vi "1D Explorer.vi"() -> ()   [LabVIEW 2023]
doc: "Demonstrates how to find the roots, maxima, and minima points for an equation entered on the front panel. This example also finds the integral and derivative for the equation."
uses:
  <vilib>/gmath/NI_Gmath.lvlib
panel:
  in  "Graph Options":i32[](listbox)
  out "Graph":cluster{dbl[], dbl[]}[](graph)
  out "error":i32
  in  "formula":string="sinc(c)+sin(2*c)+sin(3*c)+sin(2*c*c)"
  in  "Stop":bool
  in  "start":dbl format="%#.6g"
  in  "end":dbl=4.0 format="%#.6g"
  in  "# of points":u32=32
  # "Overview: Demonstrates the use of the symbolic functions.\nRequirements: LabVIEW Full Development System\nInstructions:\n1. Run the VI.\n2. Select different Graph Options and observe the results in the Graph. Note that you can Ctrl-click items in the list to display multiple plots at once.\n3. Click Stop to stop the VI."
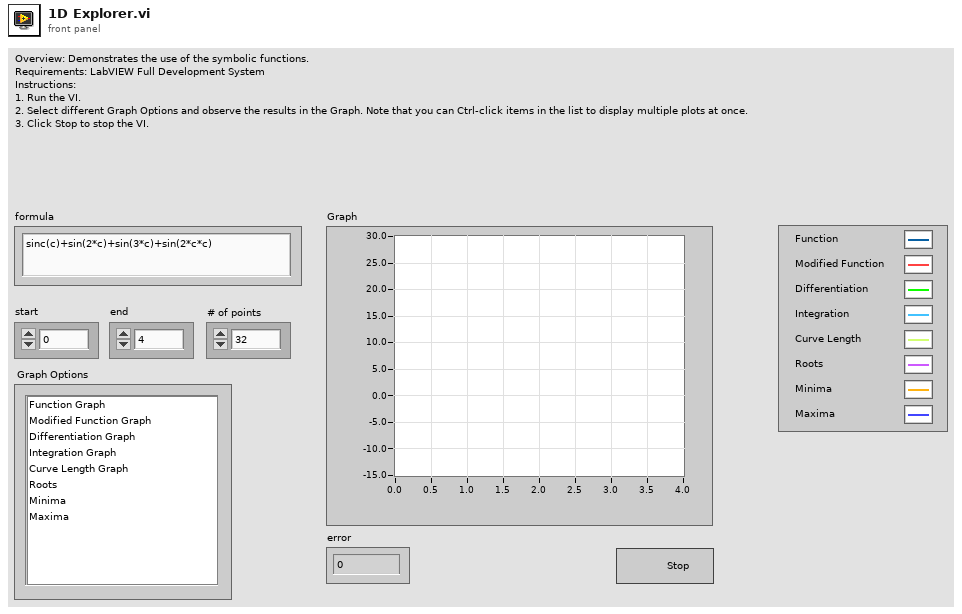
[diagram p1: front panel]
types:
  T1 = cluster{"X Values":dbl[], "Derivative of Y":dbl[]}
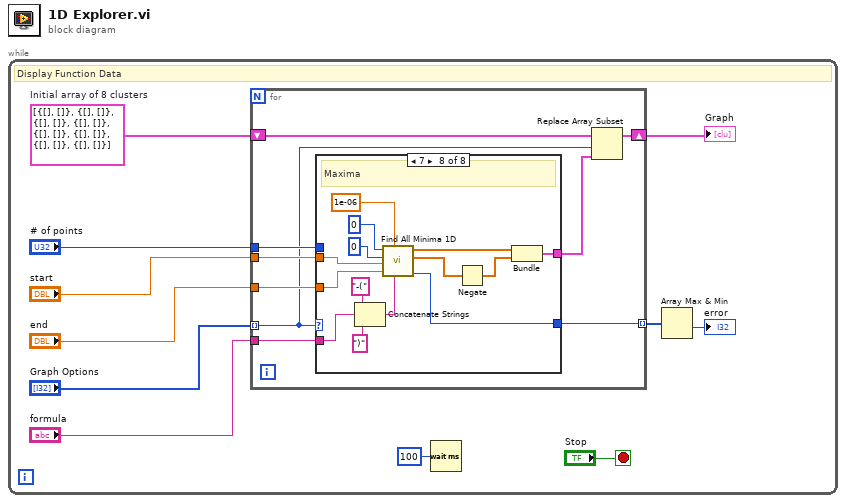
[diagram p0: block diagram]
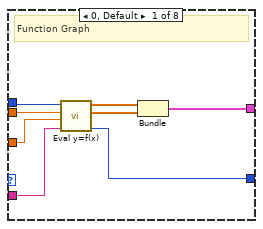
[diagram p2: hidden frame]
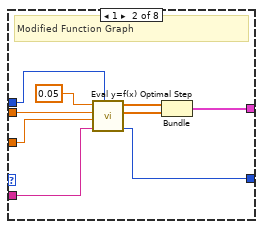
[diagram p3: hidden frame]
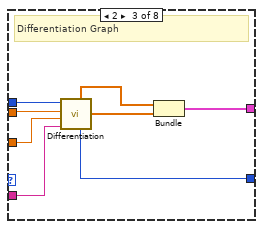
[diagram p4: hidden frame]
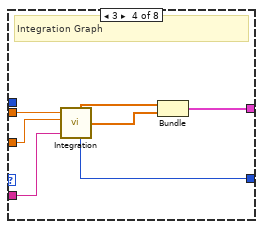
[diagram p5: hidden frame]
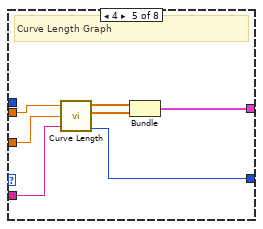
[diagram p6: hidden frame]
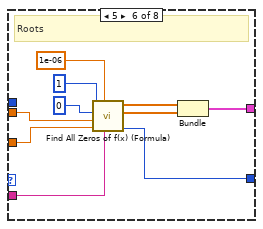
[diagram p7: hidden frame]
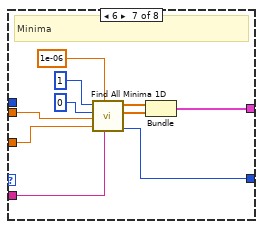
[diagram p8: hidden frame]
diagram:
  n1 = while {
    stop <- "Stop" stop-if-true
    w1 = cluster{dbl[], dbl[]}[] [{[], []}, {[], []}, {[], []}, {[], []}, {[], []}, {[], []}, {[], []}, {[], []}]  # Initial array of 8 clusters
    # "Display Function Data"
    n2 = for {
      tunnel: "Graph Options" -> [w16] mode=indexing
      tunnel: "# of points" -> [w20]
      tunnel: "start" -> [w19]
      tunnel: "end" -> [w18]
      tunnel: "formula" -> [w17]
      shift-right: [w14] -> w9
      shift-left: w1 -> [w15]
      tunnel: [w13] -> w5 mode=indexing
      n3 = case shown="7" w16 {
        tunnel: w20 -> [w28 w31 w43 _ _ _ _ _]
        tunnel: w19 -> [w27 w37 w42 w52 w59 w65 w75 w90]
        tunnel: w18 -> [w26 w36 w41 w51 w58 w64 w74 w89]
        tunnel: w17 -> [w25 w35 w45 w50 w57 w69 w79 w88]
        tunnel: [w22 w32 w44 w49 w54 w66 w76 w91] -> w12
        tunnel: [w21 w30 w38 w48 w53 w63 w73 w83] -> w13
        frame 0, Default {
          # "Function Graph"
          n4 = call <vilib>:"Eval y=f(x).vi"("formula"=w25, "end"=w26, "start"=w27, "number of points"=w28) -> ("error"=w21:i32, "Y Values"=w23:dbl[], "X Values"=w24:dbl[])  [unwired: 1 out]
          n5 = Bundle("X Values"=w24, "Y Values"=w23) -> (w22:cluster{"X Values":dbl[], "Y Values":dbl[]})  [unwired: 1 in]
        }
        frame 1 {
          # "Modified Function Graph"
          n6 = call <vilib>:"Eval y=f(x) Optimal Step.vi"("number of points"=w31, "formula"=w35, "end"=w36, "start"=w37, "epsilon"=0.05) -> ("error"=w30:i32, "Y Values"=w33:dbl[], "X Values"=w34:dbl[])  [unwired: 1 out]
          n7 = Bundle("X Values"=w34, "Y Values"=w33) -> (w32:cluster{"X Values":dbl[], "Y Values":dbl[]})  [unwired: 1 in]
        }
        frame 2 {
          # "Differentiation Graph"
          n8 = call <vilib>:"Differentiation.vi"("formula"=w45, "end"=w41, "start"=w42, "number of points"=w43) -> ("error"=w38:i32, "Derivative of Y"=w39:dbl[], "X Values"=w40:dbl[])  [unwired: 2 out]
          n9 = Bundle("X Values"=w40, "Derivative of Y"=w39) -> (w44:T1)  [unwired: 1 in]
        }
        frame 3 {
          # "Integration Graph"
          n10 = call <vilib>:"Integration.vi"("formula"=w50, "end"=w51, "start"=w52) -> ("error"=w48:i32, "Integral of Y"=w46:dbl[], "X Values"=w47:dbl[])  [unwired: 2 out]
          n11 = Bundle("X Values"=w47, "Integral of Y"=w46) -> (w49:cluster{"X Values":dbl[], "Integral of Y":dbl[]})  [unwired: 1 in]
        }
        frame 4 {
          # "Curve Length Graph"
          n12 = call <vilib>:"Curve Length.vi"("start"=w59, "end"=w58, "formula"=w57) -> ("X Values"=w56:dbl[], "Curve Length"=w55:dbl[], "error"=w53:i32)  [unwired: 1 out]
          n13 = Bundle("X Values"=w56, "Curve Length"=w55) -> (w54:cluster{"X Values":dbl[], "Curve Length":dbl[]})  [unwired: 1 in]
        }
        frame 5 {
          # "Roots"
          n14 = call <vilib>:"Find All Zeros of f(x) (Formula).vi"("formula"=w69, "accuracy"=1e-06, "end"=w64, "start"=w65, "algorithm"=0, "step type"=1) -> ("error"=w63:i32, "f(Zeros)"=w67:dbl[], "Zeros"=w68:dbl[])  [unwired: 2 in, 1 out]
          n15 = Bundle("Zeros"=w68, "f(Zeros)"=w67) -> (w66:cluster{"Zeros":dbl[], "f(Zeros)":dbl[]})  [unwired: 1 in]
        }
        frame 6 {
          # "Minima"
          n16 = call <vilib>:"Find All Minima 1D.vi"("formula"=w79, "accuracy"=1e-06, "end"=w74, "start"=w75, "algorithm"=0, "step type"=1) -> ("error"=w73:i32, "f(Minima)"=w77:dbl[], "Minima"=w78:dbl[])  [unwired: 1 out]
          n17 = Bundle("Minima"=w78, "f(Minima)"=w77) -> (w76:cluster{"Minima":dbl[], "f(Minima)":dbl[]})  [unwired: 1 in]
        }
        frame 7 {
          # "Maxima"
          n18 = Concatenate Strings("-(", w88, ")") -> (w85:string)
          n19 = call <vilib>:"Find All Minima 1D.vi"("formula"=w85, "accuracy"=1e-06, "end"=w89, "start"=w90, "algorithm"=0, "step type"=0) -> ("error"=w83:i32, "f(Minima)"=w92:dbl[], "Minima"=w93:dbl[])  [unwired: 1 out]
          n20 = Negate(x=w92) -> (-x=w84:dbl[])
          n21 = Bundle("Minima"=w93, w84) -> (w91:cluster{"Minima":dbl[], dbl[]})  [unwired: 1 in]
        }
      }
      n22 = Replace Array Subset(array=w15, new element=w12, index=w16) -> (w14:cluster{dbl[], dbl[]}[])
    }
    "Graph" <- w9
    n23 = Wait (ms)(milliseconds to wait=u32 100) -> ()  [unwired: 1 out]
    n24 = Array Max & Min(array=w5) -> (min value=→"error":i32)  [unwired: 3 out]
  }
